vi "Exchange Param.vi"(8 "error in (no error)":errorcluster, 9 "PAR":dbl[](array[numeric]), 10 "AOP":dbl[][](array[numeric]), 11 "Regs":refnum<class "bronkhorst_reg_1.lvclass">[](array[class])) -> (0 "error out":errorcluster, 3 "Regs out":refnum<class "bronkhorst_reg_1.lvclass">[](array[class]))   [LabVIEW 2019, in "bronkhorst_reg_1.lvclass"]
uses:
  bronkhorst_reg_1.lvclass
  bronkhorst_reg_1.lvclass/bronkhorst_reg_1.ctl
  Inputs/Ctl/AOParamColumns.ctl
  ctl/control param.ctl
  control.lvlib
  Inputs/Inputs.lvlib
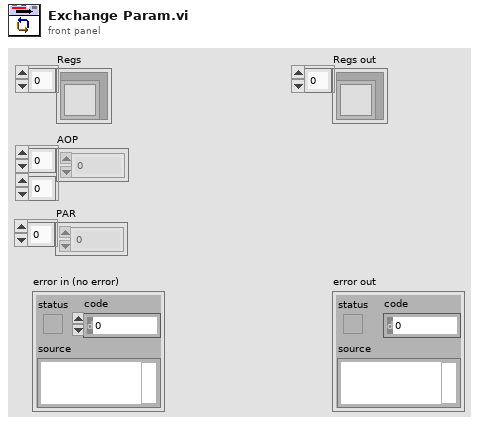
[diagram p1: front panel]
types:
  T1 = typedef "Inputs.lvlib/AOParamColumns.ctl" = enum16{"instrument_gain", "instrument_offset", "instrument_range_min", "instrument_range_max", "output_pv_min", "output_pv_max", "output_register_min", "output_register_max", "module_fcode_full", "control_channel_num", "fcode", "fcodef", "fcode_full", "fname", "instrument_units"}
  T2 = typedef "control.lvlib/control param.ctl" = cluster{"proportional gain (Kc)":dbl, "integral time (Ti, s)":dbl, "derivative time (Td, s)":dbl, "output high":dbl, "output high start":dbl, "output high stop":dbl, "alr value":dbl, "output low":dbl, "output rate (EGU/s)":dbl, "setpoint max":dbl, "setpoint rate (EGU/min)":dbl, "stop rate (EGU/min)":dbl}
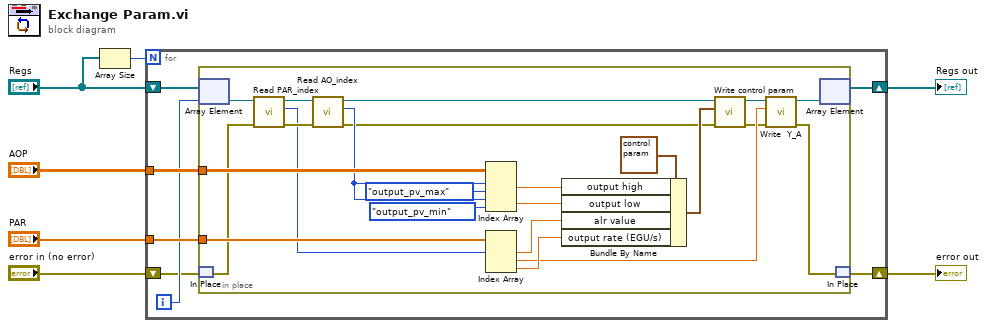
[diagram p0: block diagram]
diagram:
  n1 = Array Size(array="Regs") -> (size(s)=w2:i32)
  n2 = for {
    N: w2 -> [_]
    tunnel: "AOP" -> [w14]
    tunnel: "PAR" -> [w13]
    shift-right: [w10] -> w7
    shift-left: "Regs" -> [w12]
    shift-right: [w8] -> w3
    shift-left: "error in (no error)" -> [w9]
    i -> [w11]
    n3 = in-place {
      in-place-border: w14 -> [w37]
      in-place-border: w13 -> [w36]
      n4 = in-place-array #1(w12, w11) -> (w18:refnum<class "bronkhorst_reg_1.lvclass">)
      n5 = in-place-match #2(w9) -> (w16:errorcluster)
      n6 = call "Read PAR_index.vi"("error in (no error)"=w16, "bronkhorst_reg in"=w18) -> ("error out"=w22:errorcluster, "PAR_index"=w21:u16, "bronkhorst_reg out"=w23:refnum<class "bronkhorst_reg_1.lvclass">)  [unwired: 7 in]
      n7 = call "Read AO_index.vi"("error in (no error)"=w22, "bronkhorst_reg in"=w23) -> ("error out"=w20:errorcluster, "AO_index"=w24:u16, "bronkhorst_reg out"=w25:refnum<class "bronkhorst_reg_1.lvclass">)  [unwired: 7 in]
      n8 = Index Array(array=w37, index (row) #1=w24, index (col) #1=AOParamColumns."output_pv_max" ("AOParamColumns"), index (row) #2=w24, index (col) #2=AOParamColumns."output_pv_min" ("AOParamColumns")) -> (element #1=w34:dbl, element #2=w33:dbl)
      n9 = Index Array(array=w36, index #1=w21) -> (element #1=w32:dbl, element #2=w26:dbl, element #3=w28:dbl)  [unwired: 2 in]
      n10 = Bundle By Name(cluster=T2 {"proportional gain (Kc)"=1.0, "integral time (Ti, s)"=10.0, "derivative time (Td, s)"=1.0, "output high"=100.0, "output high start"=40.0, "output high stop"=40.0, "alr value"=0.0, "output low"=0.0, "output rate (EGU/s)"=5.0, "setpoint max"=100.0, "setpoint rate (EGU/min)"=10.0, "stop rate (EGU/min)"=5.0} ("control param"), "output high"=w34, "output low"=w33, "alr value"=w32, "output rate (EGU/s)"=w28) -> (w31:T2)
      n11 = call "Write control param.vi"("error in (no error)"=w20, "control param"=w31, "reg in"=w25) -> ("error out"=w19:errorcluster, "reg out"=w27:refnum<class "bronkhorst_reg_1.lvclass">)  [unwired: 7 in]
      n12 = call "Write  Y_A.vi"("error in (no error)"=w19, "Y_A"=w26, "reg in"=w27) -> ("error out"=w15:errorcluster, "reg out"=w17:refnum<class "bronkhorst_reg_1.lvclass">)  [unwired: 7 in]
      n13 = in-place-array #1(w17) -> (w10:refnum<class "bronkhorst_reg_1.lvclass">[])  [unwired: 1 out]
      n14 = in-place-match #2(w15) -> (w8:errorcluster)
    }
  }
  "error out" <- w3
  "Regs out" <- w7
